vi "SendMsg.vi"(1 "Body":u8[](array[numeric]), 3 "Length":u16, 4 "ID":u8) -> ()   [LabVIEW 2016]
uses:
  SndMsgType.ctl
  GlobalVars.vi
panel:
  out "Msg Len":u16
  out "Out Msg Idx":u16
  out "Out Msg":u8[](array[numeric])
  out "Msg":u8[](array[numeric])
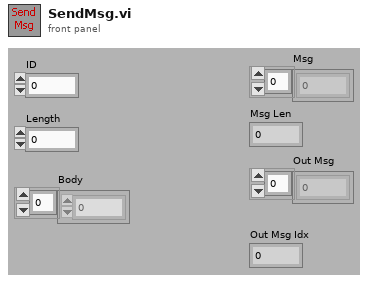
[diagram p1: front panel]
types:
  T1 = typedef "SndMsgType.ctl" = cluster{"Length":u16, "Formatted Msg":u8[]}
  T2 = typedef "Queue RefNum" = refnum<k1>
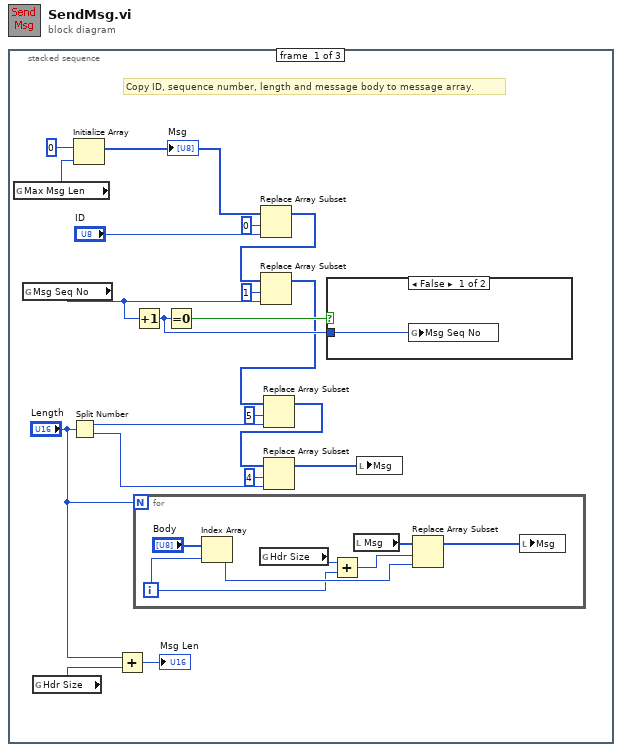
[diagram p0: block diagram]
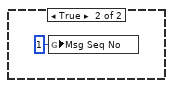
[diagram p2: hidden frame]
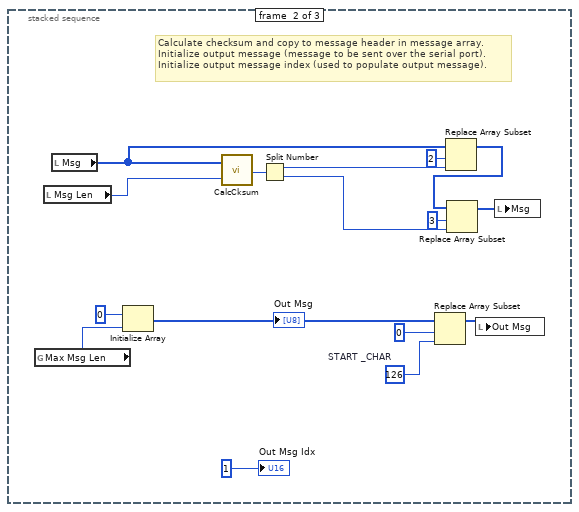
[diagram p3: hidden frame]
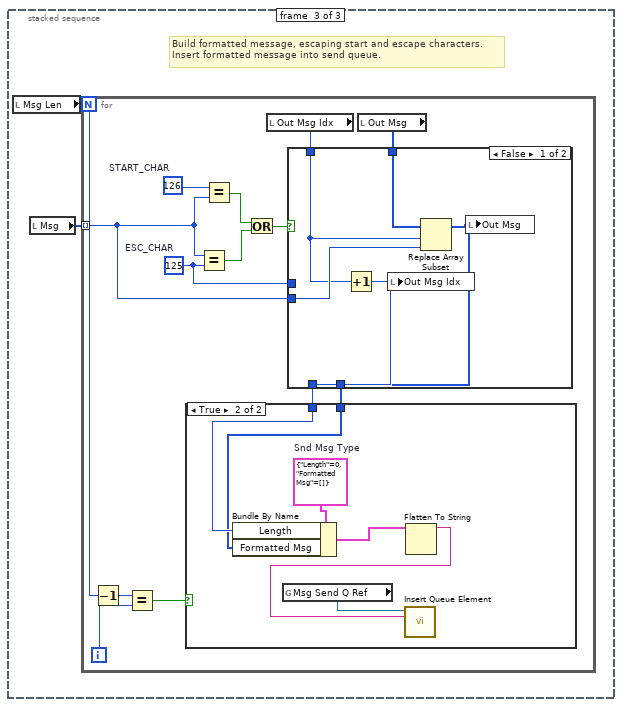
[diagram p4: hidden frame]
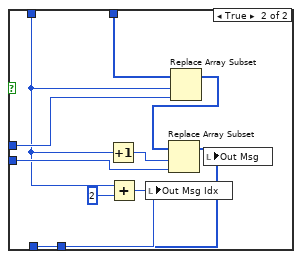
[diagram p6: hidden frame]
diagram:
  n1 = stacked-sequence {
    frame #0 {
      # "Copy ID, sequence number, length and message body to message array."
      n2 = global read "GlobalVars.vi" "Max Msg Len"() -> (w19:u16)
      n3 = global read "GlobalVars.vi" "Msg Seq No"() -> (w15:u8)
      n4 = global read "GlobalVars.vi" "Hdr Size"() -> (w7:u8)
      n5 = Split Number(x="Length") -> (hi(x)=w10:u8, lo(x)=w9:u8)
      n6 = Initialize Array "Initialize Array"(u8 0 ("Element Data"), w19) -> (w5:u8[])
      "Msg" <- w5
      n7 = Add(x="Length", y=w7) -> (x+y=→"Msg Len":u16)
      n8 = Increment(x=w15) -> (x+1=w13:u8)
      n9 = for {
        N: "Length" -> [_]
        i -> [w24]
        n10 = Index Array "Index Array"(array="Body", index=w24) -> (element=w27:u8)
        n11 = global read "GlobalVars.vi" "Hdr Size"() -> (w25:u8)
        n12 = Add(x=w25, y=w24) -> (x+y=w23:i32)
        n13 = local read "Msg"() -> (w22:u8[])
        n14 = Replace Array Subset "Replace Array Subset"(array=w22, new element=w27, index=w23) -> (w21:u8[])
        n15 = local write "Msg"(w21) -> ()
      }
      n16 = Equal To 0?(x=w13) -> (x = 0?=w14:bool)
      n17 = Replace Array Subset "Replace Array Subset"(array=w5, new element="ID", index=0 ("Index")) -> (w4:u8[])
      n18 = Replace Array Subset "Replace Array Subset"(array=w4, new element=w15, index=1 ("Index")) -> (w3:u8[])
      n19 = Replace Array Subset "Replace Array Subset"(array=w3, new element=w10, index=5 ("Index")) -> (w2:u8[])
      n20 = Replace Array Subset "Replace Array Subset"(array=w2, new element=w9, index=4 ("Index")) -> (w1:u8[])
      n21 = case shown="False" w14 {
        tunnel: w13 -> [w28 _]
        frame False {
          n22 = global write "GlobalVars.vi" "Msg Seq No"(w28) -> ()
        }
        frame True {
          n23 = global write "GlobalVars.vi" "Msg Seq No"(u8 1 ("Msg Seq No")) -> ()
        }
      }
      n24 = local write "Msg"(w1) -> ()
    }
    frame #1 {
      w35 = u8 126  # START _CHAR
      # "Calculate checksum and copy to message header in message array.\nInitialize output message (message to be sent over the serial port).\nInitialize output message index (used to populate output message)."
      n25 = global read "GlobalVars.vi" "Max Msg Len"() -> (w38:u16)
      n26 = local read "Msg Len"() -> (w34:u16)
      n27 = local read "Msg"() -> (w33:u8[])
      n28 = Initialize Array "Initialize Array"(u8 0 ("Element Data"), w38) -> (w37:u8[])
      "Out Msg" <- w37
      n29 = call "CalcCksum.vi"("Byte Cnt"=w34, "Buffer"=w33) -> ("CkSum"=w45:u16)
      n30 = Split Number(x=w45) -> (hi(x)=w42:u8, lo(x)=w41:u8)
      n31 = Replace Array Subset "Replace Array Subset"(array=w37, new element=w35, index=0 ("Index")) -> (w30:u8[])
      n32 = Replace Array Subset "Replace Array Subset"(array=w33, new element=w42, index=2 ("Index")) -> (w32:u8[])
      n33 = Replace Array Subset "Replace Array Subset"(array=w32, new element=w41, index=3 ("Index")) -> (w31:u8[])
      n34 = local write "Out Msg"(w30) -> ()
      n35 = local write "Msg"(w31) -> ()
      "Out Msg Idx" <- u16 1 ("Idx")
    }
    frame #2 {
      # "Build formatted message, escaping start and escape characters.\nInsert formatted message into send queue."
      n36 = local read "Msg Len"() -> (w47:u16)
      n37 = local read "Msg"() -> (w46:u8[])
      n38 = for {
        N: w47 -> [w48]
        tunnel: w46 -> [w57] mode=indexing
        i -> [w53]
        w56 = u8 125  # ESC_CHAR
        w61 = u8 126  # START_CHAR
        n39 = Decrement(x=w48) -> (x-1=w49:i32)
        n40 = Equal?(x=w49, y=w53) -> (x = y?=w51:bool)
        n41 = Equal?(x=w57, y=w56) -> (x = y?=w59:bool)
        n42 = Equal?(x=w61, y=w57) -> (x = y?=w60:bool)
        n43 = Or(x=w60, y=w59) -> (x .or. y?=w58:bool)
        n44 = local read "Out Msg Idx"() -> (w54:u16)
        n45 = local read "Out Msg"() -> (w55:u8[])
        n46 = case shown="False" w58 {
          tunnel: w57 -> [w69 w80]
          tunnel: w56 -> [_ w81]
          tunnel: w55 -> [w72 w75]
          tunnel: w54 -> [w68 w76]
          tunnel: [w71 w77] -> w52
          tunnel: [w70 w73] -> w50
          frame False {
            n47 = Increment(x=w68) -> (x+1=w71:u16)
            n48 = local write "Out Msg Idx"(w71) -> ()
            n49 = Replace Array Subset "Replace Array Subset"(array=w72, new element=w69, index=w68) -> (w70:u8[])
            n50 = local write "Out Msg"(w70) -> ()
          }
          frame True {
            n51 = Increment(x=w76) -> (x+1=w79:u16)
            n52 = Add(x=w76, y=u16 2) -> (x+y=w77:u16)
            n53 = local write "Out Msg Idx"(w77) -> ()
            n54 = Replace Array Subset "Replace Array Subset"(array=w75, new element=w81, index=w76) -> (w74:u8[])
            n55 = Replace Array Subset "Replace Array Subset"(array=w74, new element=w80, index=w79) -> (w73:u8[])
            n56 = local write "Out Msg"(w73) -> ()
          }
        }
        n57 = case shown="True" w51 {
          tunnel: w52 -> [_ w65]
          tunnel: w50 -> [_ w64]
          frame False {
          }
          frame True {
            w66 = T1 {"Length"=0, "Formatted Msg"=[]}  # Snd Msg Type
            n58 = Bundle By Name "Bundle By Name"(cluster=w66, "Length"=w65, "Formatted Msg"=w64) -> (w63:T1)
            n59 = global read "GlobalVars.vi" "Msg Send Q Ref"() -> (w67:T2)
            n60 = Flatten To String(anything=w63) -> (data string=w62:string)  [unwired: 3 in, 2 out]
            n61 = call <vilib>:"Insert Queue Element.vi"("queue element"=w62, "queue"=w67) -> ()  [unwired: 5 in, 3 out]
          }
        }
      }
    }
  }
